vi "myRIO v1.0 Build MUX Configuration SPI.vi"(11 "Channel":T4) -> (2 "Configuration Bitmask Array":bool[][](array[boolean]), 3 "Channel Reservation List":T1)   [LabVIEW 2021]
uses:
  <vilib>/myRIO/Common/Instrument Driver Framework/myRIO v1.0/SPI/typedefs/SPI Channels Enum.ctl
  <vilib>/myRIO/Common/Instrument Driver Framework/myRIO v1.0/Resource Manager/typedefs/myRIO v1.0 Channel Reservation List.ctl
  <vilib>/myRIO/Common/Instrument Driver Framework/myRIO v1.0/Resource Manager/typedefs/myRIO v1.0 Channel Reservation Info.ctl
  <vilib>/myRIO/Common/Instrument Driver Framework/myRIO v1.0/Resource Manager/typedefs/myRIO v1.0 Connector List.ctl
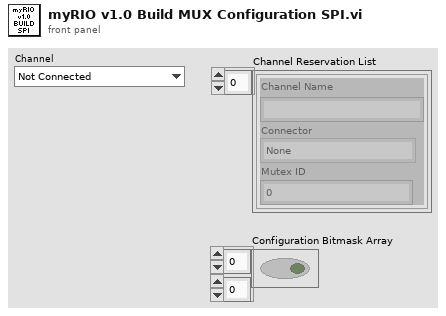
[diagram p1: front panel]
types:
  T1 = typedef "myRIO v1.0 Channel Reservation List.ctl" = T2[]
  T2 = typedef "myRIO v1.0 Channel Reservation Info.ctl" = cluster{"Channel Name":string, "Connector":T3, "Mutex ID":i32}
  T3 = typedef "myRIO v1.0 Connector List.ctl" = enum32{"None", "ConnectorA", "ConnectorB", "ConnectorC"}
  T4 = typedef "SPI Channels Enum.ctl" = enum16{"Not Connected", "A/SPI", "B/SPI", "SPI/SPI"}
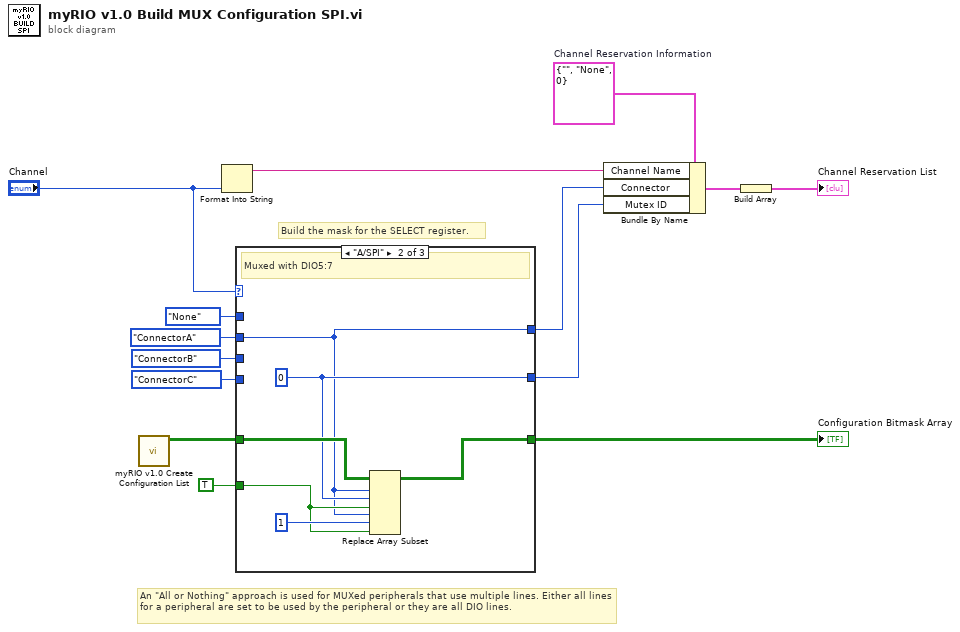
[diagram p0: block diagram]
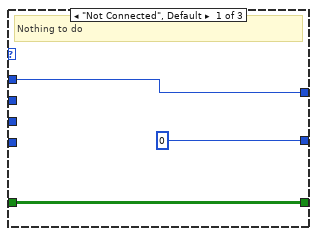
[diagram p2: hidden frame]
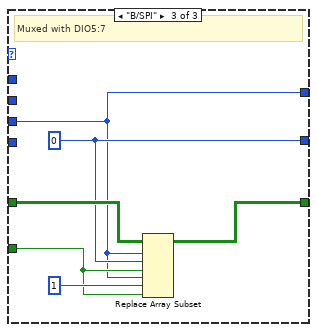
[diagram p3: hidden frame]
diagram:
  w8 = T2 {"Channel Name"="", "Connector"=enum."None", "Mutex ID"=0}  # Channel Reservation Information
  # "An \"All or Nothing\" approach is used for MUXed peripherals that use multiple lines. Either all lines for a peripheral are set to be used by the peripheral or they are all DIO lines."
  # "Build the mask for the SELECT register."
  n1 = call <vilib>:"myRIO v1.0 Create Configuration List.vi"() -> ("Bitmask Array"=w1:bool[][])  [unwired: 11 in]
  n2 = Format Into String("Channel") -> (resulting string=w7:string)  [unwired: 3 in, 1 out]
  n3 = case shown="\"A/SPI\"" "Channel" {
    tunnel: w1 -> [w17 w23 w29]
    tunnel: [w17 w22 w28] -> w11
    tunnel: myRIO_v1.0_Connector_List."None" ("Connector List") -> [w16 _ _]
    tunnel: myRIO_v1.0_Connector_List."ConnectorA" ("Connector List") -> [_ w18 _]
    tunnel: TRUE ("new element/subarray") -> [_ w19 w25]
    tunnel: myRIO_v1.0_Connector_List."ConnectorB" ("Connector List") -> [_ _ w24]
    tunnel: myRIO_v1.0_Connector_List."ConnectorC" ("Connector List") -> [_ _ _]
    tunnel: [0 ("index") w21 w27] -> w2
    tunnel: [w16 w18 w24] -> w3
    frame "Not Connected", Default {
      # "Nothing to do"
    }
    frame "A/SPI" {
      w21 = 0 ("index")
      # "Muxed with DIO5:7"
      n4 = Replace Array Subset(array=w23, new element #1=w19, index (row) #1=w18, index (col) #1=w21, new element #2=w19, index (row) #2=w18, index (col) #2=1 ("disabled index (col)")) -> (w22:bool[][])
    }
    frame "B/SPI" {
      w27 = 0 ("index")
      # "Muxed with DIO5:7"
      n5 = Replace Array Subset(array=w29, new element #1=w25, index (row) #1=w24, index (col) #1=w27, new element #2=w25, index (row) #2=w24, index (col) #2=1 ("disabled index (col)")) -> (w28:bool[][])
    }
  }
  "Configuration Bitmask Array" <- w11
  n6 = Bundle By Name(cluster=w8, "Channel Name"=w7, "Connector"=w3, "Mutex ID"=w2) -> (w6:T2)
  n7 = Build Array(w6) -> (→"Channel Reservation List":T2[])
